vi "Process TWM result.vi"(8 "error from TWM get result":errorcluster, 9 "Calculate RMS from samples":bool, 10 "TWM result":T1[][](array[typedef])) -> (0 "error out":errorcluster, 3 "TWM result as string for XCL":string[][](array[string]))   [LabVIEW 2020]
doc: "Obtain TWM result. If no calculation set, result is N/A. If calculation error, result is Err."
uses:
  external libraries/TWM-1.8.7.0-client/TWM Client Quantity Record.ctl
  external libraries/TWM-1.8.7.0-client/TWM Client.lvlib
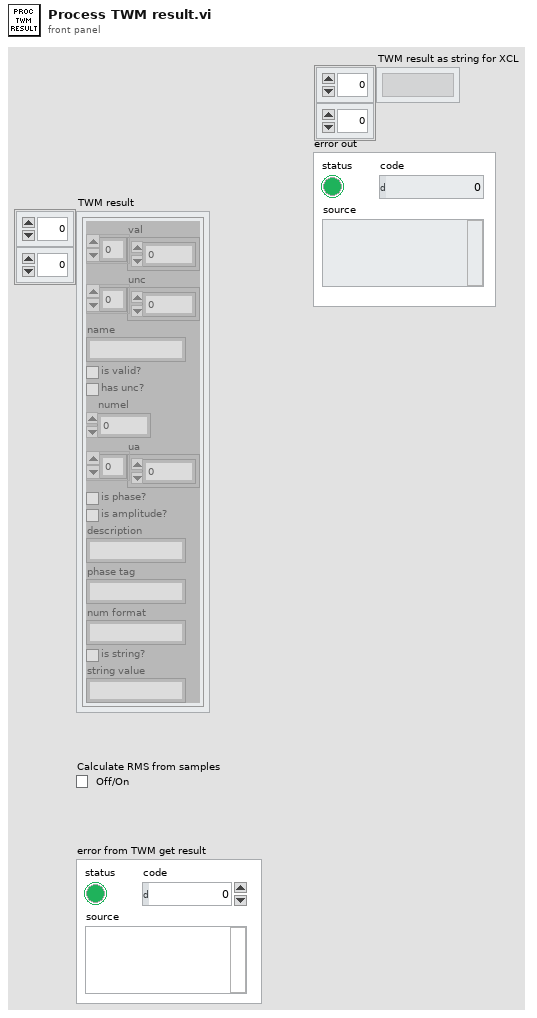
[diagram p1: front panel]
types:
  T1 = typedef "TWM Client.lvlib/TWM Client Quantity Record.ctl" = cluster{"val":dbl[], "unc":dbl[], "name":string, "is valid?":bool, "has unc?":bool, "numel":i32, "ua":dbl[], "is phase?":bool, "is amplitude?":bool, "description":string, "phase tag":string, "num format":string, "is string?":bool, "string value":string}
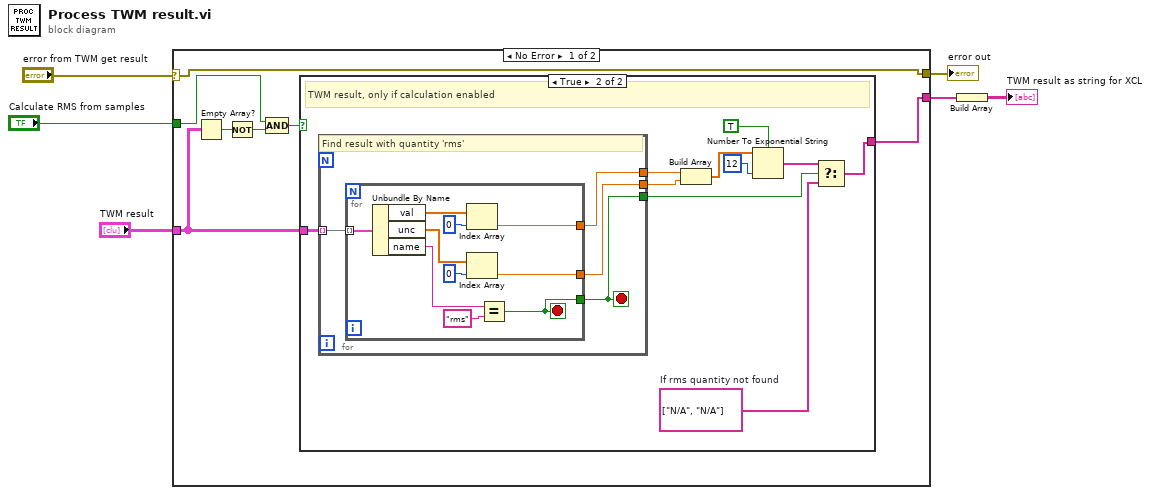
[diagram p0: block diagram]
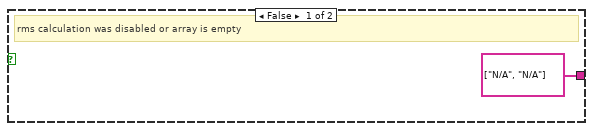
[diagram p2: hidden frame]
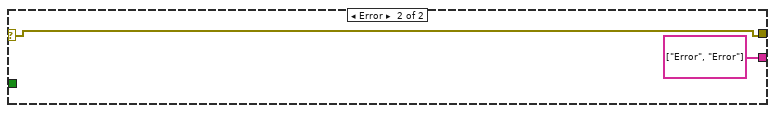
[diagram p3: hidden frame]
diagram:
  n1 = case shown="No Error" "error from TWM get result" {
    selector: "error from TWM get result" -> [w7 w39]
    tunnel: "Calculate RMS from samples" -> [w10 _]
    tunnel: "TWM result" -> [w12 _]
    tunnel: [w13 string[] ["Error", "Error"] ("f")] -> w4
    tunnel: [w7 w39] -> w2
    frame No Error {
      n2 = Empty Array?(array=w12) -> (empty?=w9:bool)
      n3 = Not(x=w9) -> (.not. x?=w8:bool)
      n4 = Compound Arithmetic op=AND(w10, w8) -> (w11:bool)
      n5 = case shown="True" w11 {
        tunnel: w12 -> [_ w24]
        tunnel: [string[] ["N/A", "N/A"] ("f") w15] -> w13
        frame False {
          # "rms calculation was disabled or array is empty"
        }
        frame True {
          w16 = string[] ["N/A", "N/A"]  # If rms quantity not found
          # "TWM result, only if calculation enabled"
          n6 = for {
            tunnel: w24 -> [w28] mode=indexing
            tunnel: [w27] -> w22
            tunnel: [w26] -> w23
            tunnel: [w25] -> w17
            stop <- w25 stop-if-true
            # "Find result with quantity 'rms'"
            n7 = for {
              tunnel: w28 -> [w38] mode=indexing
              tunnel: [w35] -> w25
              tunnel: [w33] -> w27
              tunnel: [w29] -> w26
              stop <- w35 stop-if-true
              n8 = Unbundle By Name(w38) -> ("val"=w34:dbl[], "unc"=w30:dbl[], "name"=w37:string)
              n9 = Index Array(array=w34, index=0) -> (element=w33:dbl)
              n10 = Index Array(array=w30, index=0) -> (element=w29:dbl)
              n11 = Equal?(x=w37, y="rms") -> (x = y?=w35:bool)
            }
          }
          n12 = Build Array(w22, w23) -> (w19:dbl[])
          n13 = Number To Exponential String(number=w19, precision (6)=i16 12, 1:TRUE ("use system decimal point (T)")) -> (E-format string=w18:string[])  [unwired: 1 in]
          n14 = Select(t=w18, s=w17, f=w16) -> (s? t:f=w15:string[])
        }
      }
    }
    frame Error {
    }
  }
  "error out" <- w2
  n15 = Build Array(w4) -> (→"TWM result as string for XCL":string[][])
